vi "L--C1.vi"(6 "Command Info In":T2, 8 "L--C1":T1={"1a"=0.0, "1d"=100.5, "1s"=0.8}) -> (0 "Command Info Out":T2)   [LabVIEW 2017]
uses:
  <vilib>/Rock Robotics/WPI/Framework/Command Status Info.ctl
  <vilib>/Rock Robotics/WPI/Framework/Completion Status.ctl
  <vilib>/Rock Robotics/WPI/Framework/Completion Notifier.ctl
  Block Clusters/L--C1.ctl
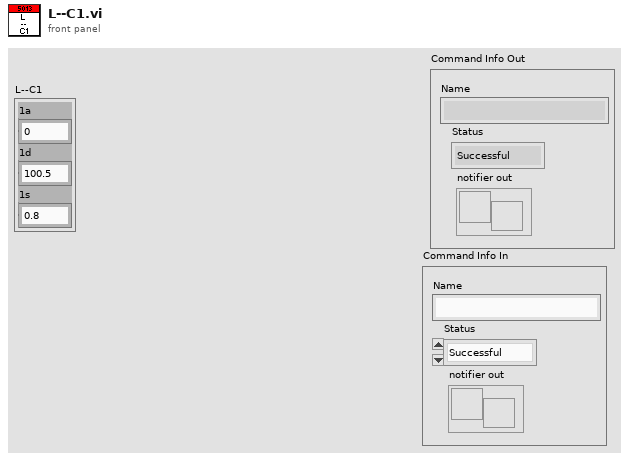
[diagram p1: front panel]
types:
  T1 = typedef "L--C1.ctl" = cluster{"1a":dbl, "1d":dbl, "1s":dbl}
  T2 = typedef "Command Status Info.ctl" = cluster{"Name":string, "Status":T3, "notifier out":T4}
  T3 = typedef "Completion Status.ctl" = enum16{"Successful", "Aborted", "Incomplete"}
  T4 = typedef "Completion Notifier.ctl" = refnum<notifier>
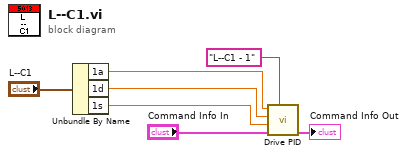
[diagram p0: block diagram]
diagram:
  n1 = Unbundle By Name("L--C1") -> ("1a"=w3:dbl, "1d"=w5:dbl, "1s"=w4:dbl)
  n2 = call "Drive PID.vi"("Description"="L--C1 - 1", "Command Info In"="Command Info In", "Speed"=w4, "Distance"=w5, "Target Angle"=w3) -> ("Command Info Out"=→"Command Info Out":T2)  [unwired: 6 in]
